vi "Log Starter.vi"(8 "error in":errorcluster, 10 "Actor-to-Caller Enqueuer":refnum<class "Message Enqueuer.lvclass">) -> (0 "error in":errorcluster, 2 "Caller-To-Actor Enqueuer":refnum<class "Message Enqueuer.lvclass">)   [LabVIEW 2012, in "Generic Instrument.lvlib" / "Generic Instrument.lvclass"]
uses:
  Generic Instrument.lvclass
  <vilib>/ActorFramework/Message Enqueuer/Message Enqueuer.lvclass
  Data Logger/Data Logger.lvclass
  <vilib>/ActorFramework/Actor/Actor.lvclass
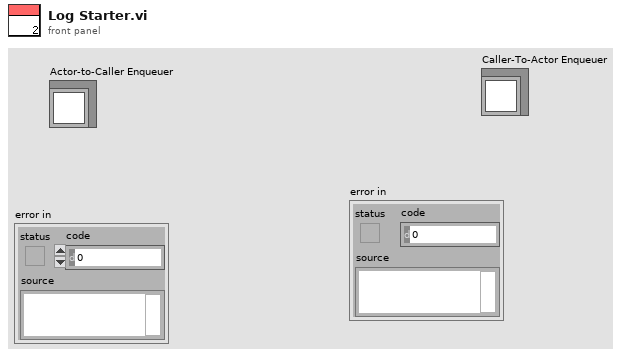
[diagram p1: front panel]
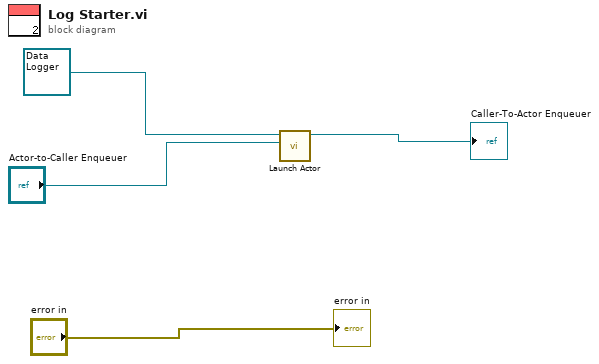
[diagram p0: block diagram]
diagram:
  n1 = call <vilib>:"Launch Actor.vi"("Actor-to-Caller Enqueuer"="Actor-to-Caller Enqueuer", "Actor"=refnum<class "Data Logger.lvclass"> refnum ("Data Logger.lvlib:Data Logger.lvclass")) -> ("Caller-To-Actor Enqueuer"=→"Caller-To-Actor Enqueuer":refnum<class "Message Enqueuer.lvclass">)  [unwired: 8 in, 1 out]
  "error in" <- "error in"
